vi "Tab Control Ref.vi"(7 "Page Label":string="Page 1", 8 "error in":errorcluster, 11 "TabControl Reference":refnum<vi>) -> (0 "error out":errorcluster, 2 "Array Out":string[](array[string]), 3 "Array":refnum<vi>[](array[refnum]))   [LabVIEW 2022 SP3]
panel:
  out "Array 2":string[](array[string])
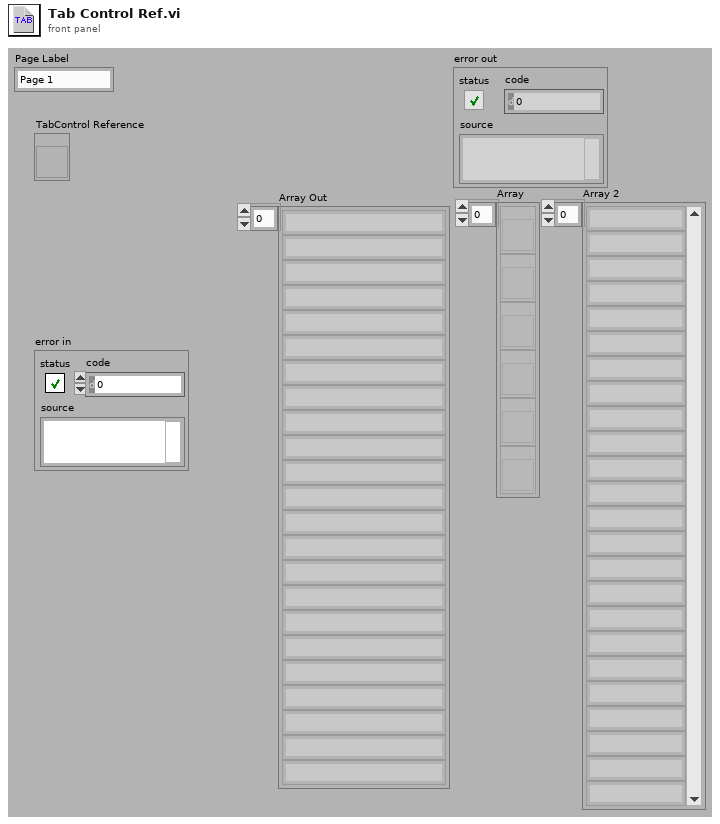
[diagram p1: front panel]
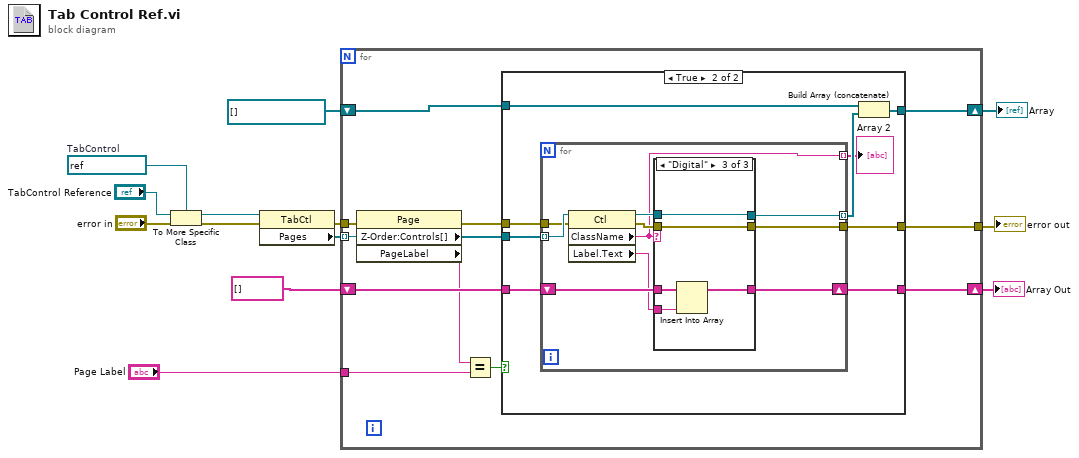
[diagram p0: block diagram]
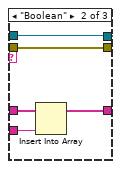
[diagram p4: hidden frame]
diagram:
  w10 = refnum<vi> refnum  # TabControl
  n1 = To More Specific Class(target class=w10, reference="TabControl Reference", error in="error in") -> (specific class reference=w8:refnum<vi>, error out=w7:errorcluster)
  n2 = property class="TabCtl"(reference=w8, error in=w7) -> (error out=w13:errorcluster, "Pages"=w11:refnum<vi>[])  [unwired: 1 out]
  n3 = for {
    tunnel: w11 -> [w25] mode=indexing
    shift-right: [w23] -> w12
    shift-left: string[] [] ("Array In") -> [w22]
    tunnel: w13 -> [w21]
    tunnel: "Page Label" -> [w18]
    tunnel: [w16] -> w5
    shift-right: [w15] -> w4
    shift-left: refnum<vi>[] [] ("Array 2") -> [w14]
    n4 = property class="Page"(reference=w25, error in=w21) -> (error out=w20:errorcluster, "Z-Order:Controls[]"=w24:refnum<vi>[], "PageLabel"=w19:string)  [unwired: 1 out]
    n5 = Equal?(x=w19, y=w18) -> (x = y?=w17:bool)
    n6 = case shown="True" w17 {
      tunnel: w24 -> [_ w37]
      tunnel: [w28 w36] -> w23
      tunnel: w22 -> [w28 w35]
      tunnel: w20 -> [w27 w34]
      tunnel: [w27 w33] -> w16
      tunnel: [w26 w30] -> w15
      tunnel: w14 -> [w26 w32]
      frame False {
      }
      frame True {
        n7 = for {
          tunnel: w37 -> [w45] mode=indexing
          shift-right: [w46] -> w36
          shift-left: w35 -> [w47]
          tunnel: w34 -> [w44]
          tunnel: [w40] -> w33
          tunnel: [w39] -> w31 mode=indexing
          tunnel: [w38] -> w29 mode=indexing
          n8 = property class="Ctl"(reference=w45, error in=w44) -> (reference out=w42:refnum<vi>, error out=w41:errorcluster, "ClassName"=w38:string, "Label.Text"=w43:string)
          n9 = case shown="\"Digital\"" w38 {
            tunnel: w47 -> [w48 w55 w60]
            tunnel: [w48 w53 w58] -> w46
            tunnel: w43 -> [_ w54 w59]
            tunnel: w42 -> [w49 w51 w56]
            tunnel: w41 -> [w50 w52 w57]
            tunnel: [w50 w52 w57] -> w40
            tunnel: [w49 w51 w56] -> w39
            frame "", Default {
            }
            frame "Boolean" {
              n10 = Insert Into Array(array=w55, new element=w54) -> (w53:string[])  [unwired: 1 in]
            }
            frame "Digital" {
              n11 = Insert Into Array(array=w60, new element=w59) -> (w58:string[])  [unwired: 1 in]
            }
          }
        }
        "Array 2" <- w29
        n12 = Build Array (concatenate)(w32, w31) -> (w30:refnum<vi>[])
      }
    }
  }
  "Array Out" <- w12
  "error out" <- w5
  "Array" <- w4
